vi "Create Progress Bar Events.vi"(8 "error in (no error)":errorcluster, 11 "SDIST in":refnum<class "NI_AB_API_DSDIST.lvclass">) -> (0 "error out":errorcluster, 2 "progressBarEvents":T1, 3 "SDIST out":refnum<class "NI_AB_API_DSDIST.lvclass">)   [LabVIEW 2020, in "NI_AB_API_DSDIST.lvclass"]
uses:
  <vilib>/AppBuilder/AB_API/DSDIST/NI_AB_API_DSDIST.lvclass
  <resource>/Framework/Providers/Common/provcom_ProgressBar_Events.ctl
  <resource>/Framework/Providers/API/mxLvBuildError.ctl
  <vilib>/AppBuilder/AB_API/SDIST/NI_AB_API_SDIST.lvclass
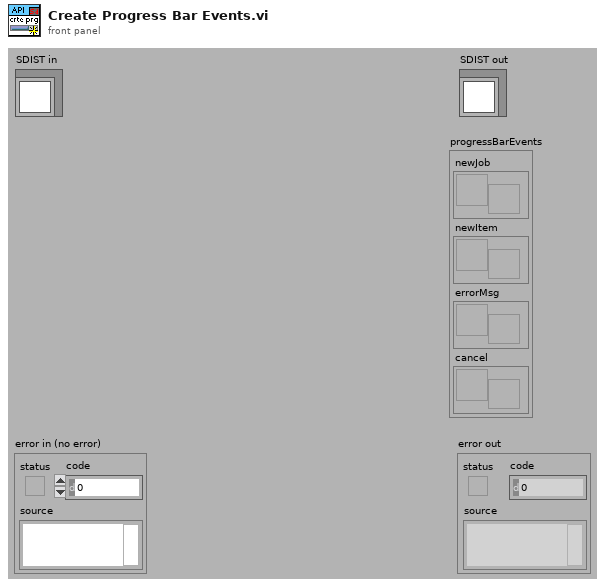
[diagram p1: front panel]
types:
  T1 = typedef "provcom_ProgressBar_Events.ctl" = cluster{"newJob":refnum<user-event>, "newItem":refnum<user-event>, "errorMsg":T2, "cancel":refnum<user-event>}
  T2 = typedef "mxLvBuildError.ctl" = refnum<user-event>
  T3 = typedef "AB_API ProgressBar_Events.ctl" = cluster{"newJob":refnum<user-event>, "newItem":refnum<user-event>, "errorMsg":T4, "cancel":refnum<user-event>}
  T4 = typedef "AB_API ProgressBar_BuildError.ctl" = refnum<user-event>
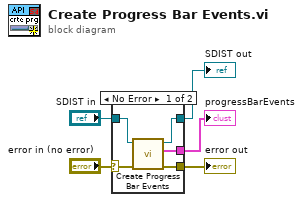
[diagram p0: block diagram]
diagram:
  n1 = case shown="No Error" "error in (no error)" {
    selector: "error in (no error)" -> [w7 w12]
    tunnel: [w6 w12] -> w4
    tunnel: [w9 w11] -> w2
    tunnel: "SDIST in" -> [w10 w11]
    tunnel: [w8 _] -> w1
    frame No Error {
      n2 = call-parent "Create Progress Bar Events.vi"("error in (no error)"=w7, "SDIST in"=w10) -> ("error out"=w6:errorcluster, "progressBarEvents"=w8:T3, "SDIST out"=w9:refnum<class "NI_AB_API_DSDIST.lvclass">)  [unwired: 7 in]
    }
    frame Error {
    }
  }
  "error out" <- w4
  "SDIST out" <- w2
  "progressBarEvents" <- w1
